vi "Read Value.vi"(8 "error in (no error)":errorcluster, 11 "fixed32 in":refnum<class "packed.lvclass">) -> (0 "error out":errorcluster, 2 "Value":refnum<class "Scalar Type.lvclass">[](array[class]), 3 "fixed32 out":refnum<class "packed.lvclass">)   [LabVIEW 2020, in "Protobuf RAW.lvlib" / "packed.lvclass"]
uses:
  packed.lvclass
  Scalar Encoder/Scalar Type.lvclass
  packed.lvclass/packed.ctl
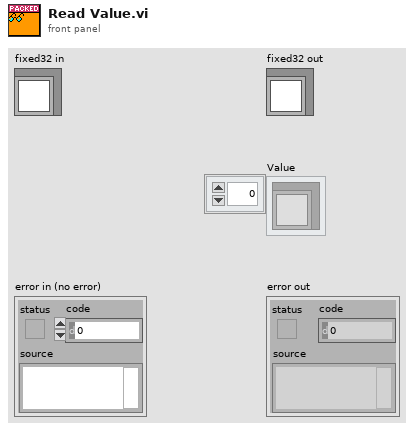
[diagram p1: front panel]
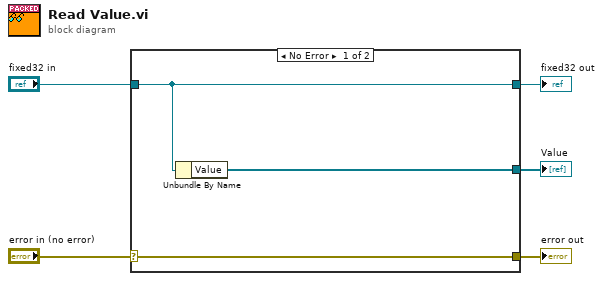
[diagram p0: block diagram]
diagram:
  n1 = case shown="No Error" "error in (no error)" {
    selector: "error in (no error)" -> [w8 w9]
    tunnel: [w8 w9] -> w4
    tunnel: [w7 w10] -> w2
    tunnel: "fixed32 in" -> [w7 w10]
    tunnel: [w6 _] -> w1
    frame No Error {
      n2 = Unbundle By Name(w7) -> ("Value"=w6:refnum<class "Scalar Type.lvclass">[])
    }
    frame Error {
    }
  }
  "error out" <- w4
  "fixed32 out" <- w2
  "Value" <- w1
